vi "fir_interpolator_test_5_25cycles.vi"() -> ()   [LabVIEW 2013]
uses:
  <vilib>/measure/maspectr.llb/Power Spectrum and PSD Export Mode.ctl
  <vilib>/measure/maspectr.llb/FFT Power Spectrum and PSD for 1 Chan.vi
  <vilib>/measure/NI_MABase.lvlib
  <vilib>/measure/NI_MAPro.lvlib
panel:
  out "Waveform Graph out":dbl[](graph)
  out "Power spectrum in":cluster{"f0":dbl, "df":dbl, "magnitude":dbl[]}(graph)
  out "Power spectrum":cluster{"f0":dbl, "df":dbl, "magnitude":dbl[]}(graph)
  out "Waveform Graph":dbl[](graph)
  out "# of Iterations":i32
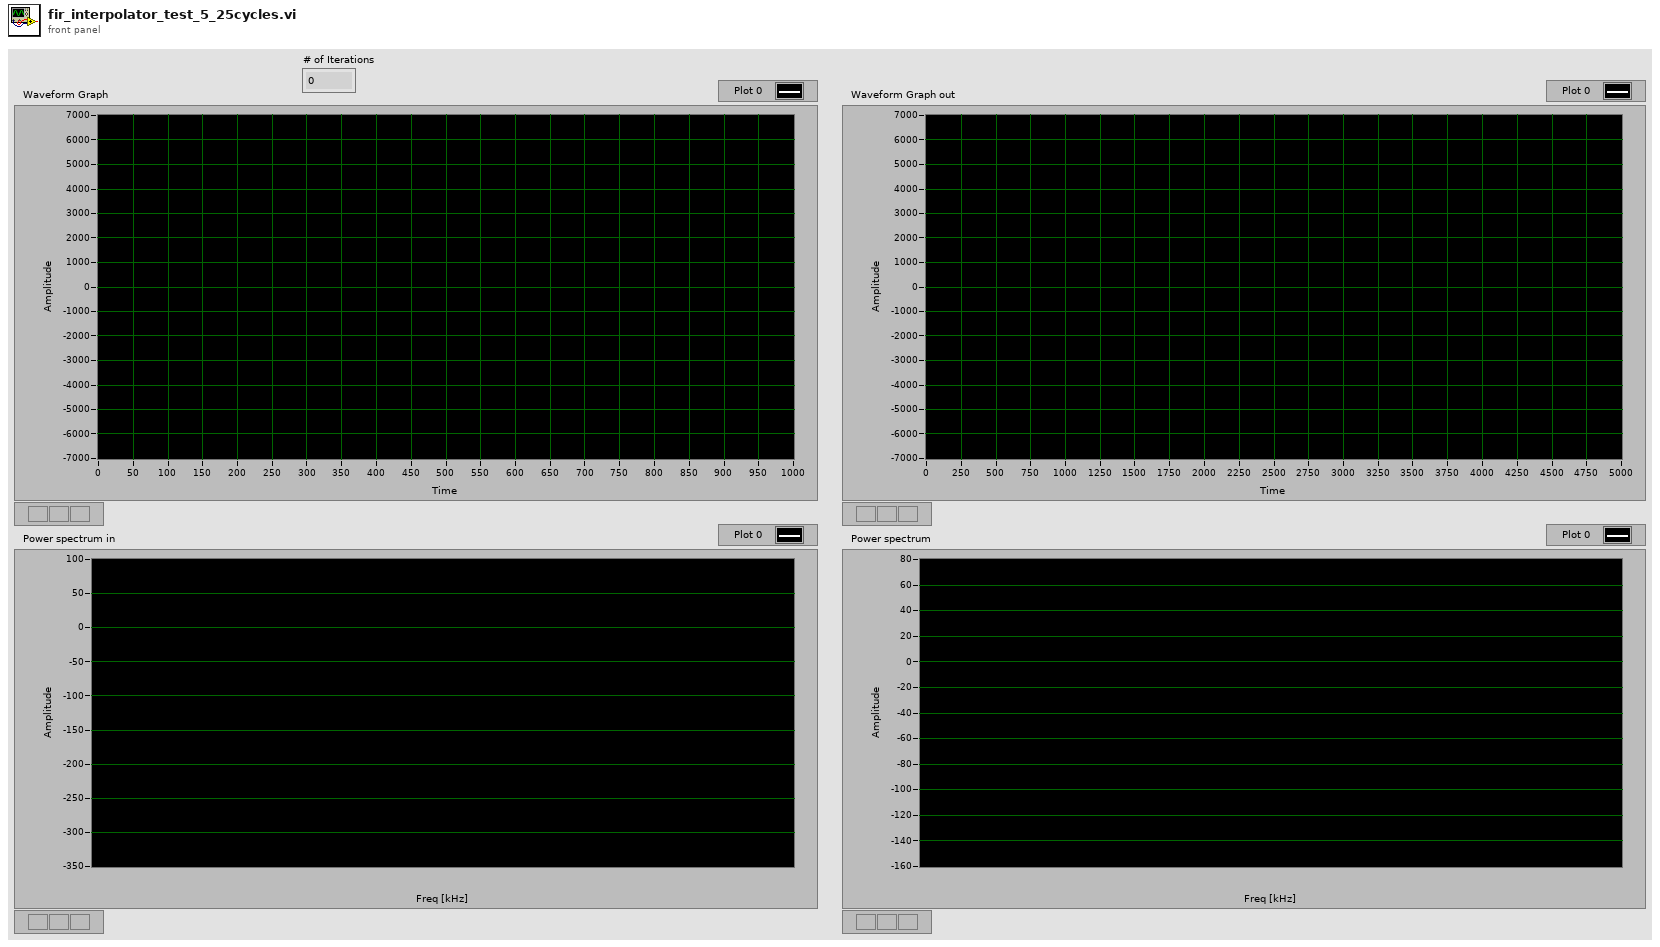
[diagram p1: front panel]
types:
  T1 = typedef "NI_MAPro.lvlib/Power Spectrum and PSD Export Mode.ctl" = u16
  T2 = cluster{"frequency":dbl, "amplitude":dbl, "phase":dbl}[]
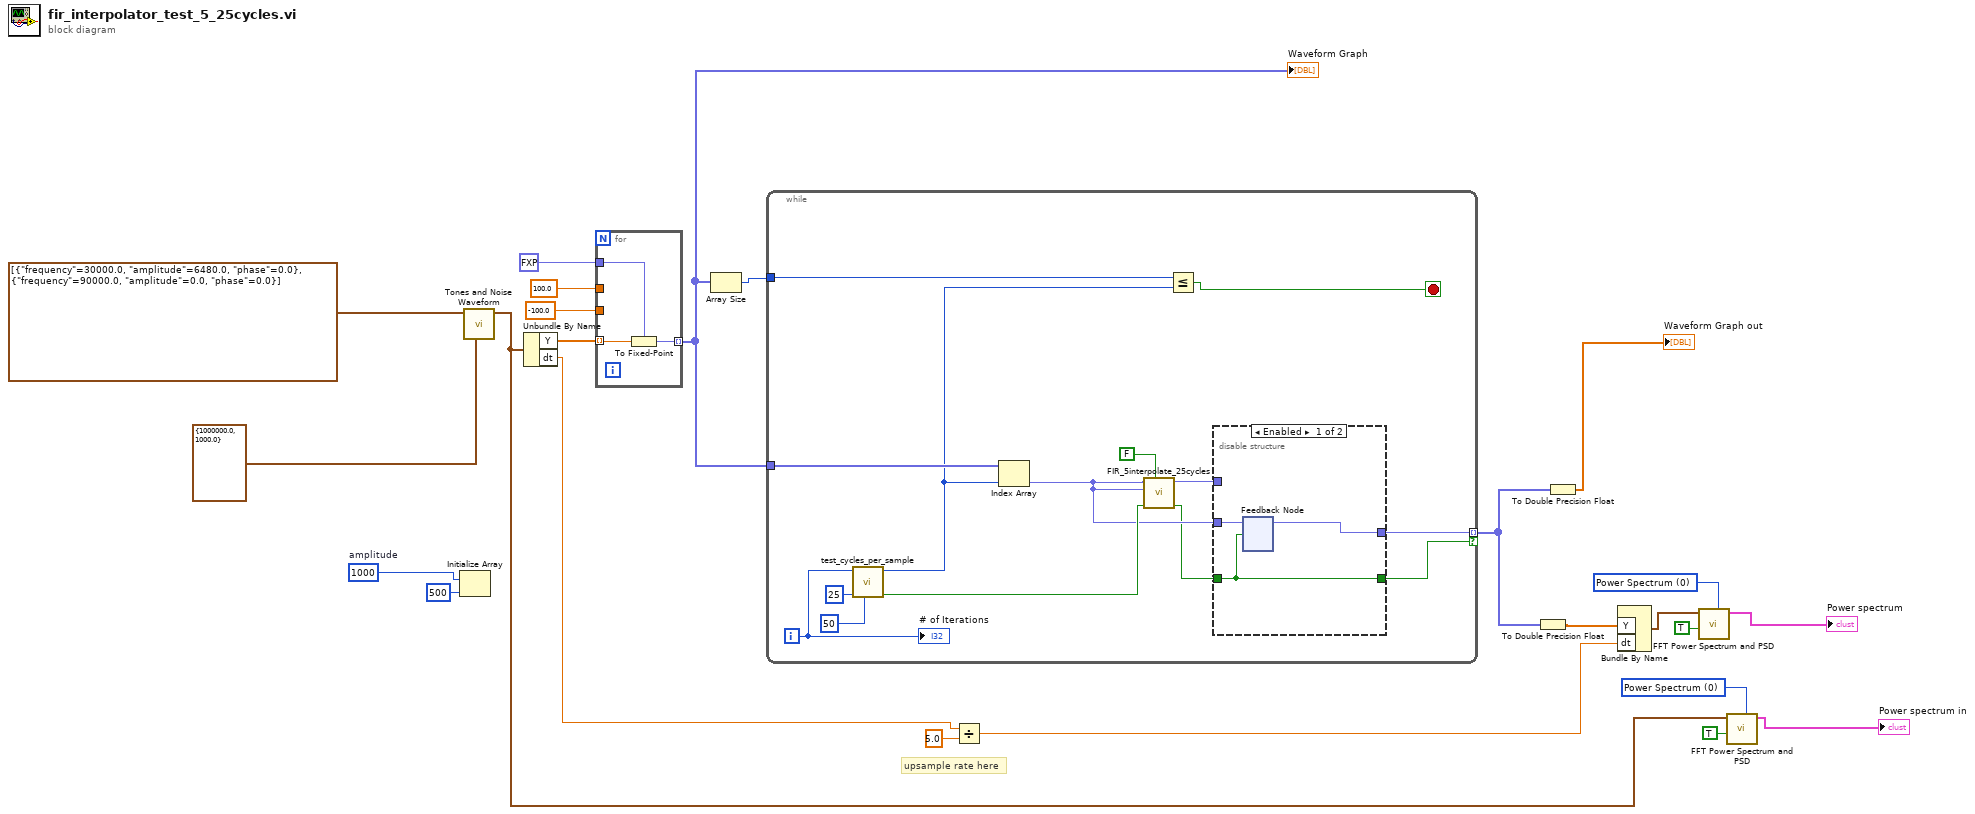
[diagram p0: block diagram]
diagram:
  w2 = 1000  # amplitude
  w12 = T1 0 items=["Power Spectrum", "Power Spectral Density"] ("export mode")
  w20 = T1 0 items=["Power Spectrum", "Power Spectral Density"] ("export mode")
  # "upsample rate here"
  n1 = Initialize Array(w2, 500 ("dimension size")) -> ()  [unwired: 1 out]
  n2 = call <vilib>:"Tones and Noise Waveform.vi"("sampling info"=cluster{"Fs":dbl, "#s":dbl} {"Fs"=1000000.0, "#s"=1000.0}, "tones"=T2 [{"frequency"=30000.0, "amplitude"=6480.0, "phase"=0.0}, {"frequency"=90000.0, "amplitude"=0.0, "phase"=0.0}]) -> ("signal out"=w11:waveform(dbl))  [unwired: 8 in, 1 out]
  n3 = Unbundle By Name(w11) -> ("Y"=w1:dbl[], "dt"=w18:dbl)
  n4 = for {
    tunnel: w1 -> [w25] mode=indexing
    tunnel: fxp<+/-,16,14> 0.0 ("fixed-point type") -> [w27]
    tunnel: [w26] -> w4 mode=indexing
    tunnel: 100.0 -> [_]
    tunnel: -100.0 -> [_]
    n5 = To Fixed-Point(fixed-point type=w27, number=w25) -> (fixed-point=w26:fxp<+/-,16,14>)
  }
  "Waveform Graph" <- w4
  n6 = Array Size(array=w4) -> (size(s)=w5:i32)
  n7 = while {
    tunnel: w4 -> [w41]
    tunnel: [w29] -> w9 mode=indexing if=w30
    tunnel: w5 -> [w37]
    i -> [w40]
    stop <- w35 stop-if-true
    n8 = call "test_cycles_per_sample.vi"("initial delay"=50, "cycles per sample"=25, "index"=w40) -> ("valid out"=w33:bool, "array index"=w36:i32)  [unwired: 7 in]
    n9 = Index Array(array=w41, index=w36) -> (element=w32:fxp<+/-,16,14>)
    n10 = call "FIR_5interpolate_25cycles.vi"("reset"=FALSE, "valid in"=w33, "Q in"=w32, "I in"=w32) -> ("valid out"=w31:bool, "I out"=w28:fxp<+/-,16,14>)  [unwired: 4 in, 2 out]
    n11 = Less Or Equal?(x=w37, y=w36) -> (x <= y?=w35:bool)
    n12 = disable-structure shown="Enabled" {
      disable-tunnel: w32 -> [w44 _]
      disable-tunnel: w31 -> [w43 w45]
      disable-tunnel: [w43 w45] -> w30
      disable-tunnel: [w42 w46] -> w29
      disable-tunnel: w28 -> [_ w46]
      frame Enabled {
        n13 = feedback-in #1(w44, w43) -> ()
        n14 = feedback #1() -> (w42:fxp<+/-,16,14>)  [unwired: 1 in]
      }
      frame Disabled {
      }
    }
    "# of Iterations" <- w40
  }
  n15 = Divide(x=w18, y=5.0) -> (x/y=w16:dbl)
  n16 = To Double Precision Float(number=w9) -> (double precision float=w14:dbl[])
  n17 = To Double Precision Float(number=w9) -> (double precision float=→"Waveform Graph out":dbl[])
  n18 = Bundle By Name("Y"=w14, "dt"=w16) -> (w21:waveform(dbl))  [unwired: 1 in]
  n19 = call-poly <vilib>:"FFT Power Spectrum and PSD.vi"("export mode"=w20, "dB On (F)"=TRUE, "time signal"=w21) -> ("Power Spectrum / PSD"=→"Power spectrum":cluster{"f0":dbl, "df":dbl, "magnitude":dbl[]})  [unwired: 5 in, 3 out]
  n20 = call-poly <vilib>:"FFT Power Spectrum and PSD.vi"("export mode"=w12, "dB On (F)"=TRUE, "time signal"=w11) -> ("Power Spectrum / PSD"=→"Power spectrum in":cluster{"f0":dbl, "df":dbl, "magnitude":dbl[]})  [unwired: 5 in, 3 out]
